vi "convert histogram data bytes to uints.vi"(10 "data out":u8[](array[numeric])) -> (2 "uint data":u32[](array[numeric]))   [LabVIEW 2017]
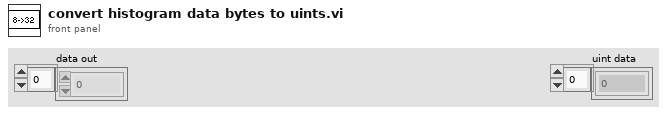
[diagram p1: front panel]
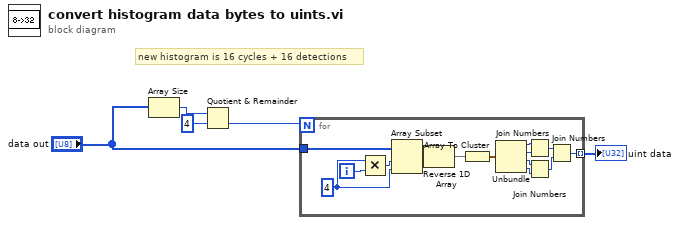
[diagram p0: block diagram]
diagram:
  # "new histogram is 16 cycles + 16 detections"
  n1 = Array Size(array="data out") -> (size(s)=w3:i32)
  n2 = Quotient & Remainder(x=w3, y=4) -> (floor(x/y)=w1:i32)  [unwired: 1 out]
  n3 = for {
    N: w1 -> [_]
    tunnel: "data out" -> [w19]
    tunnel: [w8] -> w5 mode=indexing
    i -> [w18]
    w16 = 4 ("x")
    n4 = Multiply(x=w16, y=w18) -> (x*y=w17:i32)
    n5 = Array Subset(array=w19, index=w17, length=w16) -> (w7:u8[])
    n6 = Reverse 1D Array(array=w7) -> (reversed array=w6:u8[])
    n7 = Array To Cluster(array=w6) -> (cluster=w15:cluster{"[0]":u8, "[1]":u8, "[2]":u8, "[3]":u8})
    n8 = Unbundle(w15) -> ("[0]"=w14:u8, "[1]"=w13:u8, "[2]"=w12:u8, "[3]"=w11:u8)
    n9 = Join Numbers(hi=w14, lo=w13) -> ((hi.lo)=w10:u16)
    n10 = Join Numbers(hi=w12, lo=w11) -> ((hi.lo)=w9:u16)
    n11 = Join Numbers(hi=w10, lo=w9) -> ((hi.lo)=w8:u32)
  }
  "uint data" <- w5
